vi "Write Cascade.vi"(8 "error in (no error)":errorcluster, 10 "Cascade":bool, 11 "Filter in":refnum<class "Filter.lvclass">) -> (0 "error out":errorcluster, 3 "Filter out":refnum<class "Filter.lvclass">)   [LabVIEW 2020, in "Filter.lvclass"]
uses:
  Filter.lvclass
  Filter.lvclass/Filter.ctl
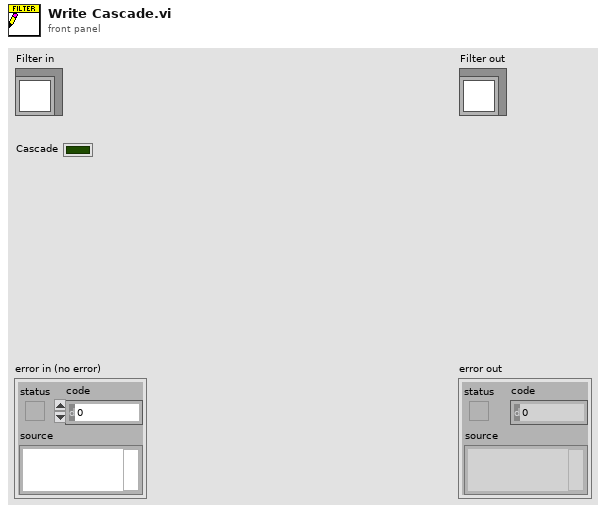
[diagram p1: front panel]
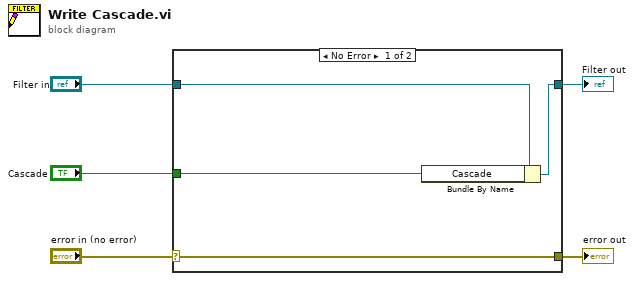
[diagram p0: block diagram]
diagram:
  n1 = case shown="No Error" "error in (no error)" {
    selector: "error in (no error)" -> [w9 w10]
    tunnel: [w9 w10] -> w4
    tunnel: [w7 w11] -> w2
    tunnel: "Filter in" -> [w8 w11]
    tunnel: "Cascade" -> [w6 _]
    frame No Error {
      n2 = Bundle By Name(cluster=w8, "Cascade"=w6) -> (w7:refnum<class "Filter.lvclass">)
    }
    frame Error {
    }
  }
  "error out" <- w4
  "Filter out" <- w2
